vi "Connect to DB.vi"(8 "error in":errorcluster, 11 "Data Cluster in":T1) -> (0 "error out":errorcluster, 3 "Data Cluster out":T1)   [LabVIEW 2020, in "hse-db.lvlib" / "DB_CONNECTOR.lvlib"]
doc: "Establish a connection to the database.\n\n<b>Note:</b> This VI was modified by the <b>Validate DQMH Module</b> tool to be shared clone reentrant.\n\n____\nHAMPEL SOFTWARE ENGINEERING v1.4.0 (2023-12-19 09:52)"
uses:
  DB_CONNECTOR.lvlib
  Module Data--cluster.ctl
  DB-Interface/DB-Interface.lvclass
  hse-libraries/Source/hse-configuration/config-base/config-base.lvclass
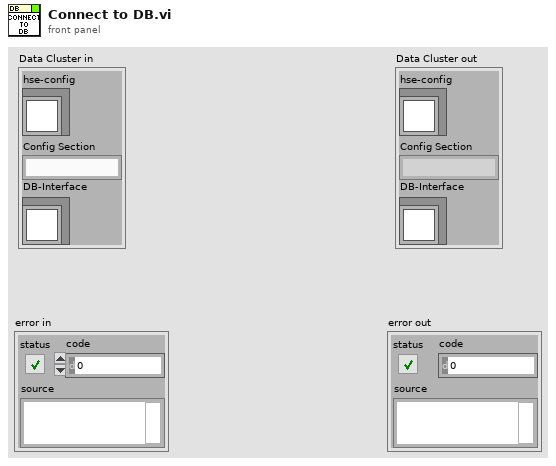
[diagram p1: front panel]
types:
  T1 = typedef "hse-db.lvlib/DB_CONNECTOR.lvlib/Module Data--cluster.ctl" = cluster{"hse-config":refnum<class "config-base.lvclass">, "Config Section":string, "DB-Interface":refnum<class "DB-Interface.lvclass">}
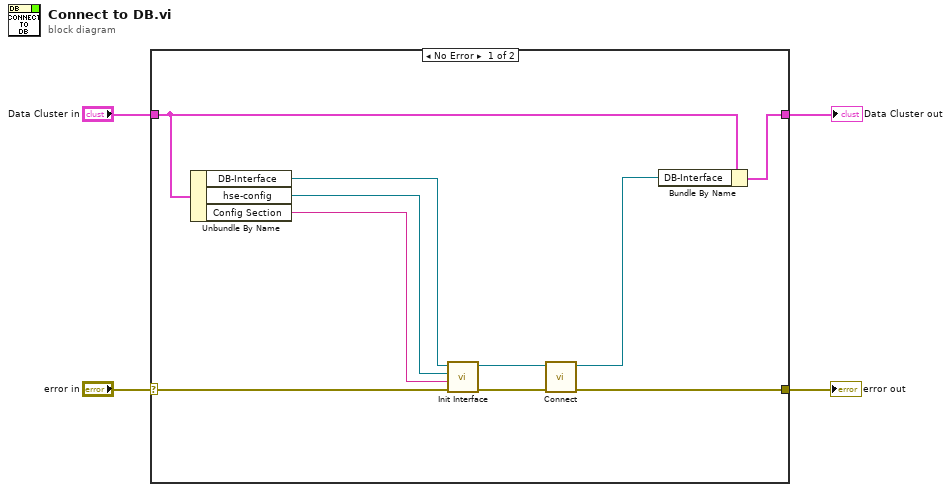
[diagram p0: block diagram]
diagram:
  n1 = case shown="No Error" "error in" {
    selector: "error in" -> [w12 w16]
    tunnel: [w10 w16] -> w4
    tunnel: [w14 w15] -> w3
    tunnel: "Data Cluster in" -> [w13 w15]
    frame No Error {
      n2 = Unbundle By Name(w13) -> ("DB-Interface"=w5:refnum<class "DB-Interface.lvclass">, "hse-config"=w7:refnum<class "config-base.lvclass">, "Config Section"=w6:string)
      n3 = call-dynamic "Init Interface.vi"("error in"=w12, "Config Section"=w6, "hse-config"=w7, "DB-Interface in"=w5) -> ("error out"=w11:errorcluster, "DB-Interface out"=w8:refnum<class "DB-Interface.lvclass">)  [unwired: 6 in]
      n4 = call-dynamic "Connect.vi"("error in"=w11, "DB-Engine in"=w8) -> ("error out"=w10:errorcluster, "DB-Engine out"=w9:refnum<class "DB-Interface.lvclass">)  [unwired: 8 in]
      n5 = Bundle By Name(cluster=w13, "DB-Interface"=w9) -> (w14:T1)
    }
    frame Error {
    }
  }
  "error out" <- w4
  "Data Cluster out" <- w3
